vi "Finalize To Settings.vi"(8 "error in (no error)":errorcluster, 11 "Configuration in":refnum<class "Configuration.lvclass">) -> (0 "error out":errorcluster, 2 "settings":cluster{"key":string, "value":string}[](array[cluster]), 3 "Configuration out":refnum<class "Configuration.lvclass">)   [LabVIEW 2020, in "DSF Core.lvlib" / "Configuration.lvclass"]
uses:
  Configuration.lvclass
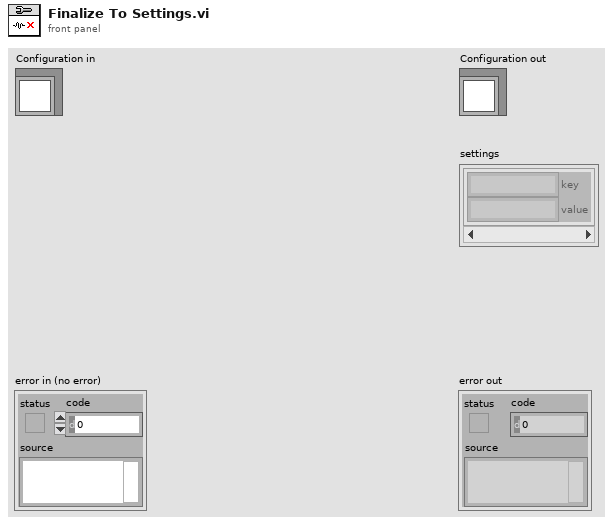
[diagram p1: front panel]
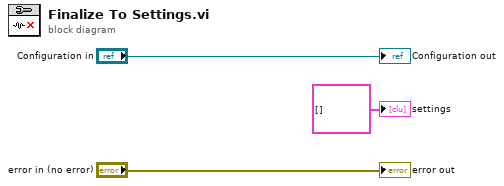
[diagram p0: block diagram]
diagram:
  "error out" <- "error in (no error)"
  "Configuration out" <- "Configuration in"
  "settings" <- cluster{"key":string, "value":string}[] [] ("settings")
